vi "avgOfTwoNumbers2.vi"() -> ()   [LabVIEW 2021]
panel:
  out "Result":dbl
  in  "B":dbl
  in  "A":dbl
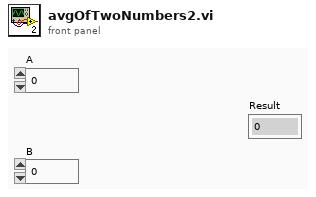
[diagram p1: front panel]
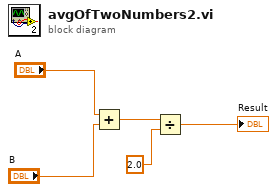
[diagram p0: block diagram]
diagram:
  n1 = Add(x="A", y="B") -> (x+y=w3:dbl)
  n2 = Divide(x=w3, y=2.0) -> (x/y=→"Result":dbl)
